vi "Move to filter position.vi"(6 "Skip cell?":bool, 9 "Filter Wheel Positions":dbl[][](array[numeric])=[[0.0, 0.0], [1.0, 30.0], [2.0, 60.0], [3.0, 90.0], [4.0, 120.0], [5.0, 150.0], [6.0, 240.0], [7.0, 270.0], [8.0, 300.0], [9.0, 330.0], [10.0, 207.5]], 10 "Current anlge (degrees)":dbl, 11 "Filter no.":dbl) -> (0 "error out":errorcluster, 4 "New current anlge (degrees)":dbl)   [LabVIEW 2016]
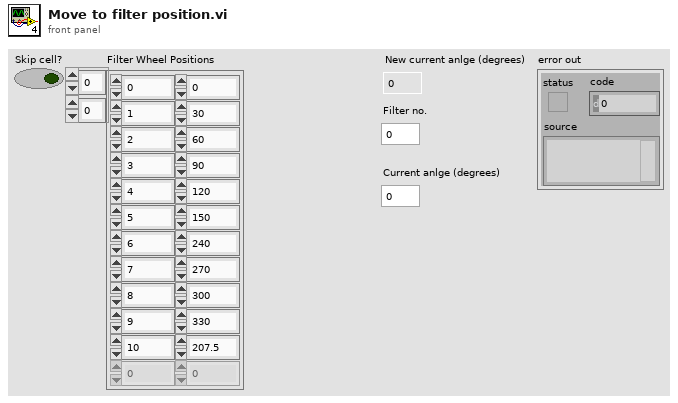
[diagram p1: front panel]
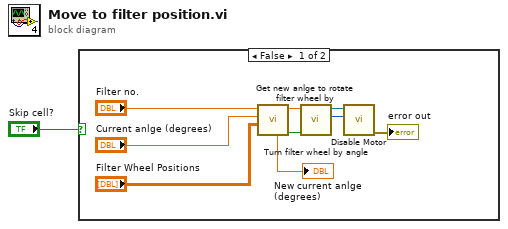
[diagram p0: block diagram]
diagram:
  n1 = case shown="False" "Skip cell?" {
    frame False {
      n2 = call "Get new anlge to rotate filter wheel by.vi"("Filter Wheel Positions"="Filter Wheel Positions", "Current anlge (degrees)"="Current anlge (degrees)", "Filter no."="Filter no.") -> ("Clockwise?"=w7:bool, "Rotate by angle (degrees)"=w8:dbl, "New current anlge (degrees)"=→"New current anlge (degrees)":dbl)  [unwired: 6 in]
      n3 = call "Turn filter wheel by angle.vi"("Clockwise?"=w7, "Angle (degrees)"=w8) -> ("Enable Channel out"=w10:u8, "Serial Port out"=w9:refnum<visa-resource-name>)  [unwired: 7 in, 1 out]
      n4 = call "Disable Motor.vi"("Enable Channel"=w10, "Serial Port"=w9) -> ("error out"=→"error out":errorcluster)  [unwired: 9 in]
    }
    frame True {
    }
  }
